vi "OPCWrite.vi"() -> ()   [LabVIEW 2021]
panel:
  out "Simulated Temp":dbl
  in  "stop temp sim":bool
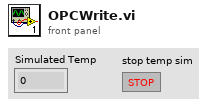
[diagram p1: front panel]
types:
  T1 = enum16{"Read", "Write", "ReadWrite", "BufferedRead", "BufferedReadWrite"}
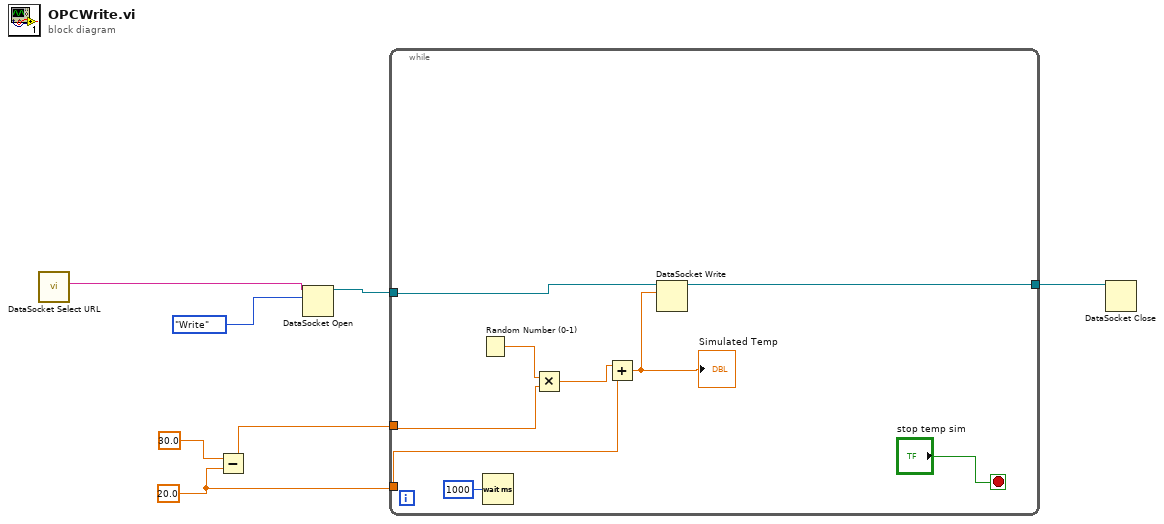
[diagram p0: block diagram]
diagram:
  w1 = 20.0
  n1 = call <vilib>:"DataSocket Select URL.vi"() -> ("URL"=w4:string)  [unwired: 9 in, 2 out]
  n2 = Subtract(x=30.0, y=w1) -> (x-y=w2:dbl)
  n3 = DataSocket Open(10:T1."Write" ("mode"), 11:w4) -> (3:w7:refnum<k13>)  [unwired: 2 in, 1 out]
  n4 = while {
    tunnel: w7 -> [w8]
    tunnel: [w14] -> w5
    tunnel: w2 -> [w13]
    tunnel: w1 -> [w11]
    stop <- "stop temp sim" stop-if-true
    n5 = Random Number (0-1)() -> (number: 0 to 1=w12:dbl)
    n6 = Wait (ms)(milliseconds to wait=u32 1000) -> ()  [unwired: 1 out]
    n7 = Multiply(x=w12, y=w13) -> (x*y=w10:dbl)
    n8 = Add(x=w10, y=w11) -> (x+y=w9:dbl)
    "Simulated Temp" <- w9
    n9 = DataSocket Write(10:w9, 11:w8) -> (3:w14:refnum<k13>)  [unwired: 2 in, 2 out]
  }
  n10 = DataSocket Close(11:w5) -> ()  [unwired: 2 in, 2 out]
